vi "Solar Example.vi"(10 "VISA resource name 2":refnum<visa-resource-name>) -> ()   [LabVIEW 2024]
uses:
  <vilib>/Instr/_visa.llb/VISA Configure Serial Port (Instr).vi
panel:
  out "read buffer":string
  in  "stop":bool
  out "Waveform Chart":dbl(graph)
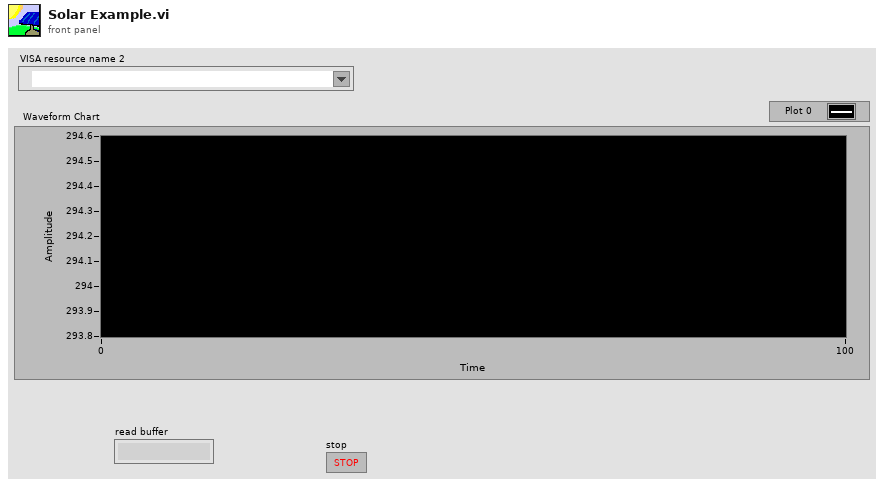
[diagram p1: front panel]
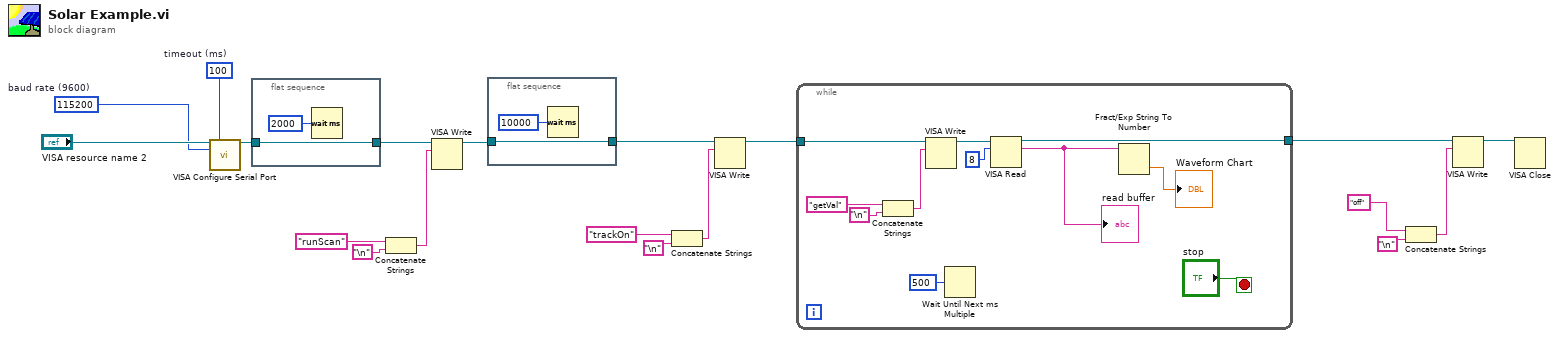
[diagram p0: block diagram]
diagram:
  w2 = u32 115200  # baud rate (9600)
  w1 = u32 100  # timeout (ms)
  n1 = call-poly "VISA Configure Serial Port"("VISA resource name"="VISA resource name 2", "timeout (10sec)"=w1, "baud rate (9600)"=w2) -> ("VISA resource name out"=w5:refnum<visa-resource-name>)  [unwired: 11 in, 1 out]
  n2 = flat-sequence {
    tunnel: w5 -> [w20]
    tunnel: [w20] -> w4
    frame #0 {
      n3 = Wait (ms)(milliseconds to wait=u32 2000) -> ()  [unwired: 1 out]
    }
  }
  n4 = Concatenate Strings("runScan" ("string"), "\n") -> (w19:string)
  n5 = VISA Write(VISA resource name=w4, write buffer=w19) -> (VISA resource name out=w16:refnum<visa-resource-name>)  [unwired: 1 in, 2 out]
  n6 = flat-sequence {
    tunnel: w16 -> [w22]
    tunnel: [w22] -> w13
    frame #0 {
      n7 = Wait (ms)(milliseconds to wait=u32 10000) -> ()  [unwired: 1 out]
    }
  }
  n8 = Concatenate Strings("trackOn" ("string"), "\n") -> (w12:string)
  n9 = VISA Write(VISA resource name=w13, write buffer=w12) -> (VISA resource name out=w11:refnum<visa-resource-name>)  [unwired: 1 in, 2 out]
  n10 = while {
    tunnel: w11 -> [w32]
    tunnel: [w26] -> w8
    stop <- "stop" stop-if-true
    n11 = Concatenate Strings("getVal" ("string"), "\n") -> (w31:string)
    n12 = VISA Write(VISA resource name=w32, write buffer=w31) -> (VISA resource name out=w30:refnum<visa-resource-name>)  [unwired: 1 in, 2 out]
    n13 = Wait Until Next ms Multiple(millisecond multiple=u32 500) -> ()  [unwired: 1 out]
    n14 = VISA Read(VISA resource name=w30, byte count=u32 8) -> (VISA resource name out=w26:refnum<visa-resource-name>, read buffer=w24:string)  [unwired: 1 in, 2 out]
    "read buffer" <- w24
    n15 = Fract/Exp String To Number(string=w24) -> (number=→"Waveform Chart":dbl)  [unwired: 3 in, 1 out]
  }
  n16 = Concatenate Strings("off" ("string"), "\n") -> (w7:string)
  n17 = VISA Write(VISA resource name=w8, write buffer=w7) -> (VISA resource name out=w6:refnum<visa-resource-name>)  [unwired: 1 in, 2 out]
  n18 = VISA Close(VISA resource name=w6) -> ()  [unwired: 1 in, 1 out]
